vi "wifiplus2Launchpad.vi"() -> ()   [LabVIEW 2012]
uses:
  Control 2.ctl
panel:
  in  "stop":bool
  in  "LED P1.6":bool
  in  "LED P1.0":T1
  out "path string":string
  out "CurrentPath":path=path "C:/Documents and Settings/TGI0362/My Documents/xUserData/LabVIEW_8.x/cmDVT_Factory-BBU-R5"
  out "new picture":picture
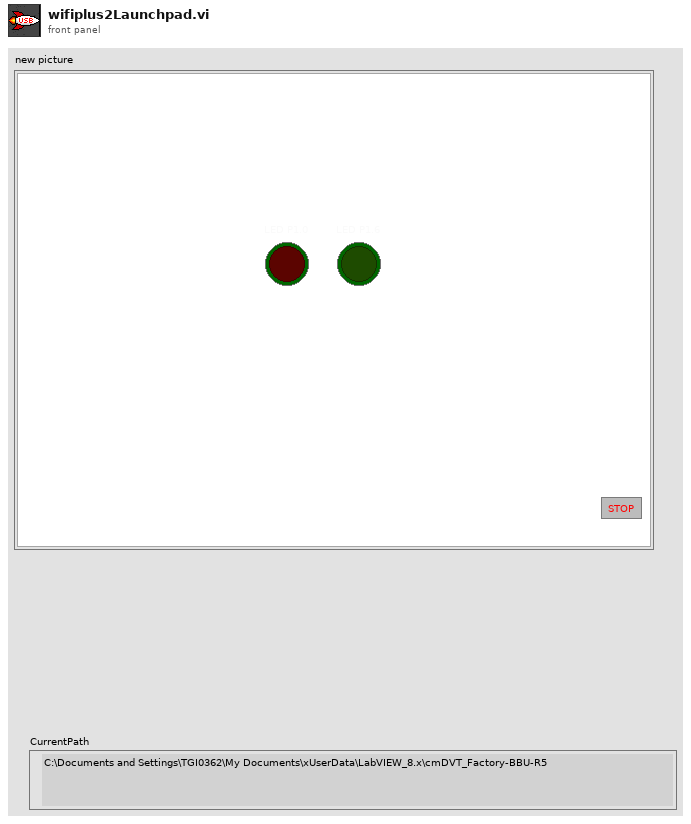
[diagram p1: front panel]
types:
  T1 = typedef "Control 2.ctl" = bool
  T2 = typedef "imagedata.ctl" = cluster{"image type":i32, "image depth":i32, "image":u8[], "mask":u8[], "colors":u32[], "Rectangle":cluster{"left":i16, "top":i16, "right":i16, "bottom":i16}}
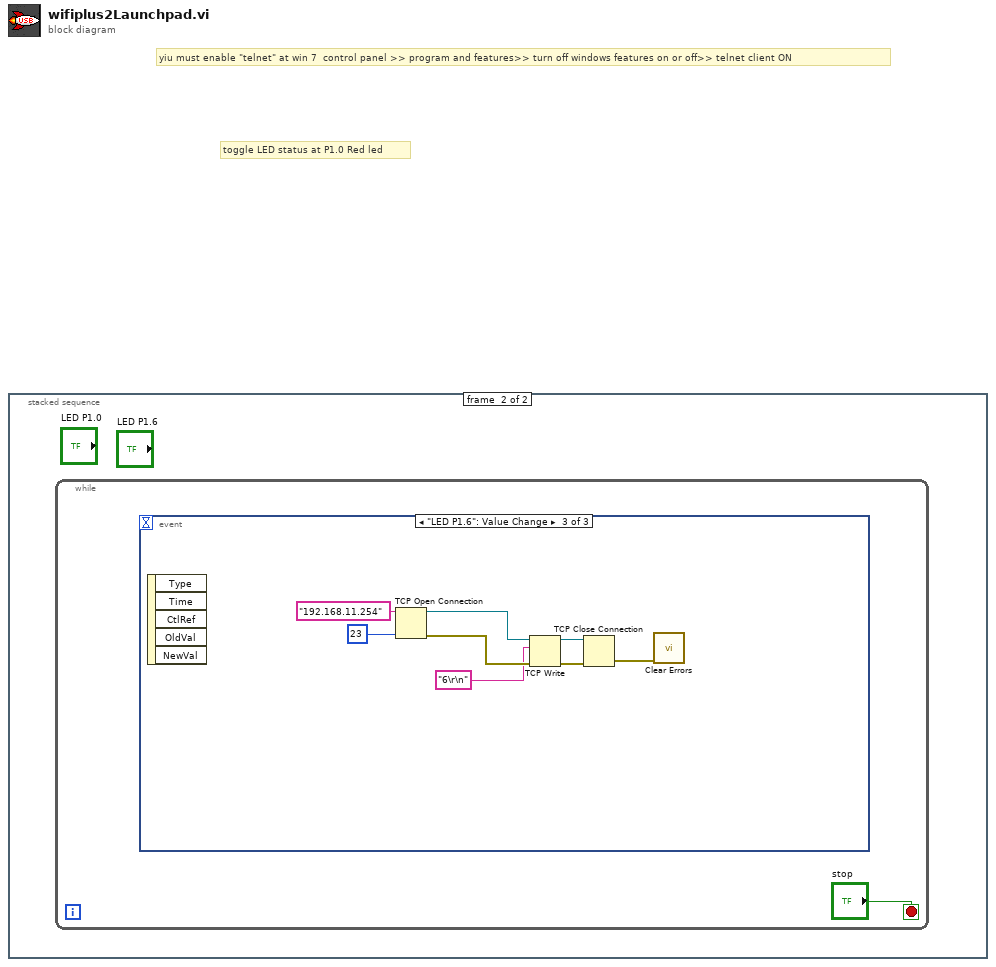
[diagram p0: block diagram]
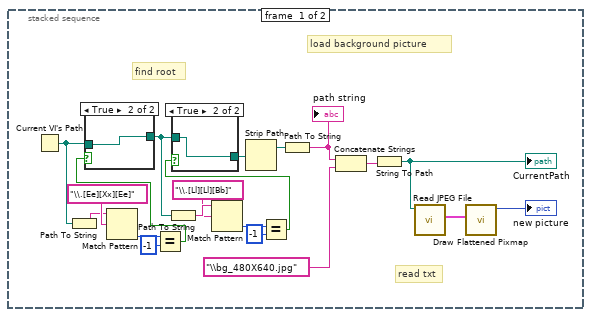
[diagram p2: hidden frame]
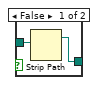
[diagram p3: hidden frame]
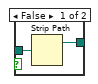
[diagram p4: hidden frame]
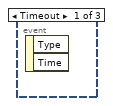
[diagram p5: hidden frame]
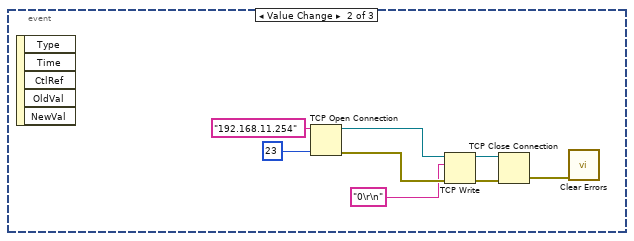
[diagram p6: hidden frame]
diagram:
  # "toggle LED status at P1.0 Red led"
  # "yiu must enable \"telnet\" at win 7  control panel >> program and features>> turn off windows features on or off>> telnet client ON"
  n1 = stacked-sequence {
    frame #0 {
      # "read txt"
      # "load background picture"
      # "find root"
      n2 = Current VI's Path() -> (path=w9:path)
      n3 = Path To String(path=w9) -> (string=w8:string)
      n4 = Match Pattern(string=w8, regular expression="\\.[Ee][Xx][Ee]") -> (offset past match=w6:i32)  [unwired: 1 in, 3 out]
      n5 = Equal?(x=w6, y=-1) -> (x = y?=w18:bool)
      n6 = case shown="True" w18 {
        tunnel: [w24 w26] -> w15
        tunnel: w9 -> [w25 w26]
        frame False {
          n7 = Strip Path(path=w25) -> (stripped path=w24:path)  [unwired: 1 out]
        }
        frame True {
        }
      }
      n8 = Path To String(path=w15) -> (string=w12:string)
      n9 = Match Pattern(string=w12, regular expression="\\.[Ll][Ll][Bb]") -> (offset past match=w14:i32)  [unwired: 1 in, 3 out]
      n10 = Equal?(x=w14, y=-1) -> (x = y?=w17:bool)
      n11 = case shown="True" w17 {
        tunnel: [w21 w23] -> w16
        tunnel: w15 -> [w22 w23]
        frame False {
          n12 = Strip Path(path=w22) -> (stripped path=w21:path)  [unwired: 1 out]
        }
        frame True {
        }
      }
      n13 = Strip Path(path=w16) -> (stripped path=w5:path)  [unwired: 1 out]
      n14 = Path To String(path=w5) -> (string=w1:string)
      "path string" <- w1
      n15 = Concatenate Strings(w1, "\\bg_480X640.jpg") -> (w3:string)
      n16 = String To Path(string=w3) -> (path=w2:path)
      "CurrentPath" <- w2
      n17 = call <vilib>:"Read JPEG File.vi"("path to JPEG file"=w2) -> ("image data"=w19:T2)  [unwired: 8 in, 2 out]
      n18 = call <vilib>:"Draw Flattened Pixmap.vi"("image data"=w19) -> ("new picture"=→"new picture":picture)  [unwired: 8 in]
    }
    frame #1 {
      n19 = while {
        stop <- "stop" stop-if-true
        n20 = event shown="[2] \"LED P1.6\": Value Change" {
          selector: _ -> [_ _ _]
          dyn-events: _ -> [_ _ _]
          timeout: _ -> [_ _ _]
          event Timeout {
            n21 = event-data() -> ()  [unwired: 1 in, 2 out]
          }
          event Value Change {
            n22 = event-data() -> ()  [unwired: 1 in, 5 out]
            n23 = TCP Open Connection(address="192.168.11.254", remote port or service name=u16 23) -> (connection ID=w33:refnum<k5>, error out=w31:errorcluster)  [unwired: 3 in]
            n24 = TCP Write(connection ID=w33, data in="0\r\n", error in (no error)=w31) -> (connection ID out=w32:refnum<k5>, error out=w30:errorcluster)  [unwired: 1 in, 1 out]
            n25 = TCP Close Connection(connection ID=w32, error in (no error)=w30) -> (error out=w29:errorcluster)  [unwired: 1 in, 1 out]
            n26 = call <vilib>:"Clear Errors.vi"("error in (no error)"=w29) -> ()  [unwired: 6 in, 1 out]
          }
          event "LED P1.6": Value Change {
            n27 = event-data() -> ()  [unwired: 1 in, 5 out]
            n28 = TCP Open Connection(address="192.168.11.254", remote port or service name=u16 23) -> (connection ID=w41:refnum<k5>, error out=w39:errorcluster)  [unwired: 3 in]
            n29 = TCP Write(connection ID=w41, data in="6\r\n", error in (no error)=w39) -> (connection ID out=w40:refnum<k5>, error out=w38:errorcluster)  [unwired: 1 in, 1 out]
            n30 = TCP Close Connection(connection ID=w40, error in (no error)=w38) -> (error out=w37:errorcluster)  [unwired: 1 in, 1 out]
            n31 = call <vilib>:"Clear Errors.vi"("error in (no error)"=w37) -> ()  [unwired: 6 in, 1 out]
          }
        }
      }
    }
  }
